vi "configureTriggering.vi"(8 "error in (no error)":errorcluster, 11 "ICCameraAcquisitor in":refnum<class "ICCameraAcquisitor.lvclass">) -> (0 "error out":errorcluster, 3 "ICCameraAcquisitor out":refnum<class "ICCameraAcquisitor.lvclass">)   [LabVIEW 2011, in "Hardware.lvlib" / "Channels.lvlib" / "ICCameraAcquisitor.lvclass"]
uses:
  ICCameraAcquisitor.lvclass
  ICCameraAcquisitor.lvclass/ICCameraAcquisitor.ctl
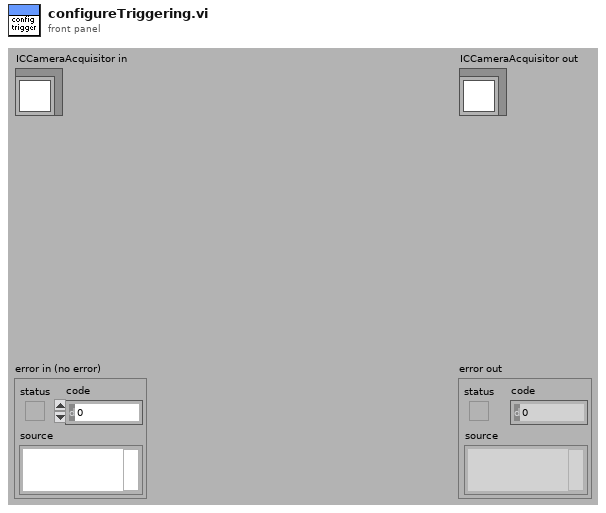
[diagram p1: front panel]
types:
  T1 = cluster{"Trigger Mode":dbl, "Fast Triggering":bool}
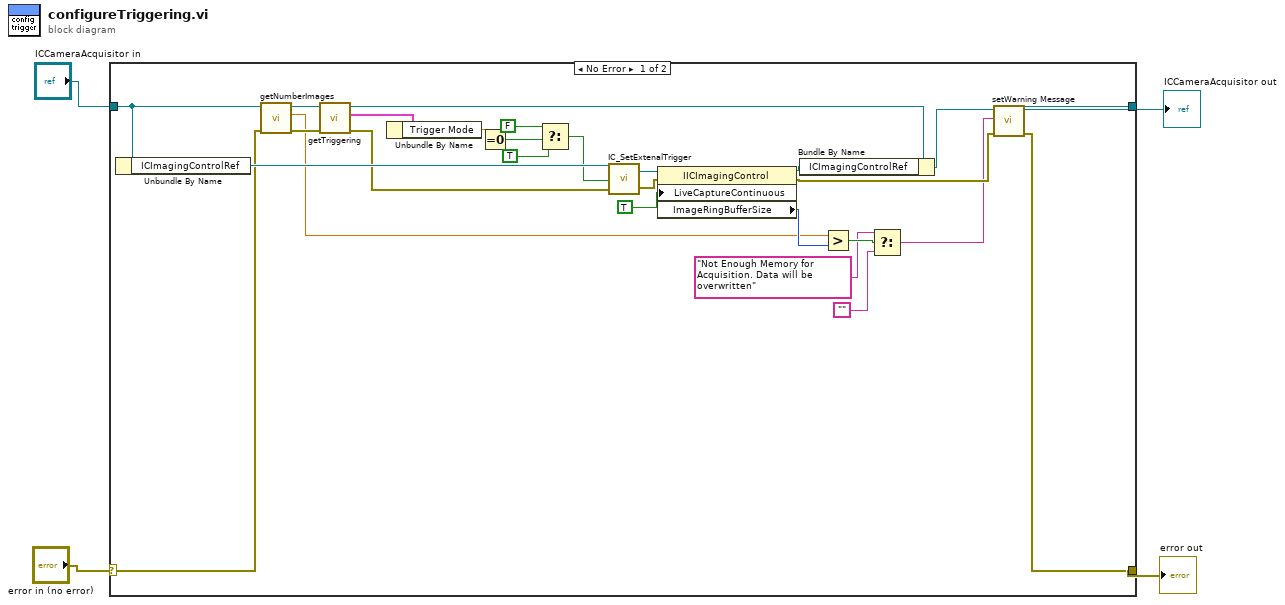
[diagram p0: block diagram]
diagram:
  n1 = case shown="No Error" "error in (no error)" {
    selector: "error in (no error)" -> [w16 w32]
    tunnel: "ICCameraAcquisitor in" -> [w18 w33]
    tunnel: [w11 w33] -> w2
    tunnel: [w6 w32] -> w1
    frame No Error {
      n2 = Unbundle By Name(w18) -> ("ICImagingControlRef"=w29:refnum<k7>)
      n3 = call-dynamic "getNumberImages.vi"("error in (no error)"=w16, "CameraAcquisitor.lvclass in"=w18) -> ("error out"=w15:errorcluster, "Number of Images"=w13:dbl, "CameraAcquisitor.lvclass out"=w17:refnum<class "ICCameraAcquisitor.lvclass">)  [unwired: 7 in]
      n4 = call-dynamic "getTriggering.vi"("error in (no error)"=w15, "CameraAcquisitor.lvclass in"=w17) -> ("error out"=w28:errorcluster, "Triggering"=w31:T1, "CameraAcquisitor.lvclass out"=w30:refnum<class "ICCameraAcquisitor.lvclass">)  [unwired: 7 in]
      n5 = Unbundle By Name(w31) -> ("Trigger Mode"=w27:dbl)
      n6 = Equal To 0?(x=w27) -> (x = 0?=w26:bool)
      n7 = Select(t=FALSE, s=w26, f=TRUE) -> (s? t:f=w23:bool)
      n8 = call <userlib>:"IC_SetExtenalTrigger.vi"("Error In (no error)"=w28, "Trigger"=w23, "ICImagingControl In"=w29) -> ("Error Out"=w19:errorcluster, "ICImagingControl Out"=w22:refnum<k7>)
      n9 = property class="IICImagingControl"(reference=w22, error in=w19, "LiveCaptureContinuous"=TRUE) -> (reference out=w21:refnum<k7>, error out=w10:errorcluster, "ImageRingBufferSize"=w14:i32)
      n10 = Bundle By Name(cluster=w30, "ICImagingControlRef"=w21) -> (w12:refnum<class "ICCameraAcquisitor.lvclass">)
      n11 = Greater?(x=w13, y=w14) -> (0:w9:bool)
      n12 = Select(t="Not Enough Memory for Acquisition. Data will be overwritten", s=w9, f="") -> (s? t:f=w7:string)
      n13 = call-dynamic "setWarning Message.vi"("error in (no error)"=w10, "Warning Message"=w7, "CameraAcquisitor.lvclass in"=w12) -> ("error out"=w6:errorcluster, "CameraAcquisitor.lvclass out"=w11:refnum<class "ICCameraAcquisitor.lvclass">)  [unwired: 7 in]
    }
    frame Error {
    }
  }
  "error out" <- w1
  "ICCameraAcquisitor out" <- w2
